vi "dvp Vi Set Awb Operation.vi"(10 "AwbOperation":u32(ring) items=["AWB_OP_OFF", "AWB_OP_ONCE", "AWB_OP_CONTINUOUS"], 11 "handle":u32) -> (3 "function return":u32(ring))   [LabVIEW 2018, in "LabViewDVPCamera.lvlib"]
doc: "LabviewDvp2Api dvpStatus dvpViSetAwbOperation(dvpHandle handle, dvpAwbOperation AwbOperation);"
uses:
  LabViewDVPCamera.lvlib
  LabViewDVPCamera/LabViewDVPCamera.dll
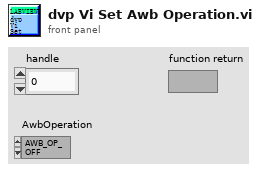
[diagram p1: front panel]
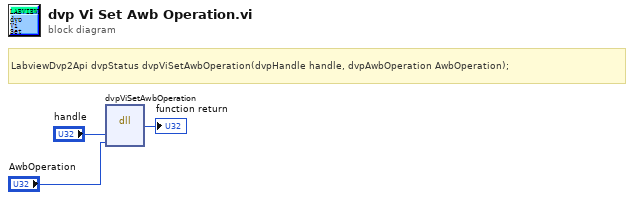
[diagram p0: block diagram]
diagram:
  # "LabviewDvp2Api dvpStatus dvpViSetAwbOperation(dvpHandle handle, dvpAwbOperation AwbOperation);"
  n1 = dll-call lib="C:/Program Files (x86)/DVP2 Labview cn 64/Sample/LabViewDVPCamera/LabViewDVPCamera.*" fn="dvpViSetAwbOperation"("handle"="handle", "AwbOperation"="AwbOperation") -> (→"function return":u32)  [unwired: 5 in, 2 out]
